vi "Sensor Loop.vi"() -> ()   [LabVIEW 2014, in "Elevator System.lvlib"]
uses:
  Elevator System.lvlib
  Typedef/FGVAction.ctl
  SimulatorVIs/Simulation Input Global.vi
  <vilib>/ptbypt/NI_PtbyPt.lvlib
panel:
  in  "elevators parameters":T1={"static gain"=10.0, "lag (s)"=0.05, "deadtime (s)"=0.01, "load"=0.0, "deadband"=0.0, "sensor noise"=0.0, "initial PV"=6.0, "plant noise"=0.0} {"plant noise" format="%.2f"; "initial PV" format="%.2f"; "sensor noise" format="%.2f"; "lag (s)" format="%.2f"; "deadtime (s)" format="%.2f"; "deadband" format="%.1f"; "load" format="%.2f"; "static gain" format="%.2f"}
  in  "gripper parameters":T1={"static gain"=2.5, "lag (s)"=2.5, "deadtime (s)"=0.01, "load"=40.0, "deadband"=0.0, "sensor noise"=0.0, "initial PV"=0.0, "plant noise"=0.0} {"plant noise" format="%.2f"; "initial PV" format="%.2f"; "sensor noise" format="%.2f"; "lag (s)" format="%.2f"; "deadtime (s)" format="%.2f"; "deadband" format="%.1f"; "load" format="%.2f"; "static gain" format="%.2f"}
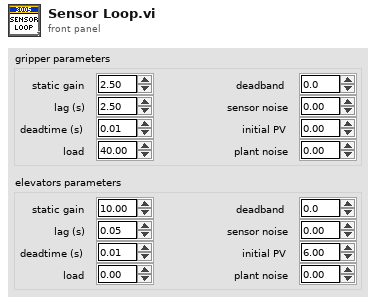
[diagram p1: front panel]
types:
  T1 = cluster{"static gain":dbl, "lag (s)":dbl, "deadtime (s)":dbl, "load":dbl, "deadband":dbl, "sensor noise":dbl, "initial PV":dbl, "plant noise":dbl}
  T2 = typedef "Elevator System.lvlib/FGVAction.ctl" = enum16{"get", "set"}
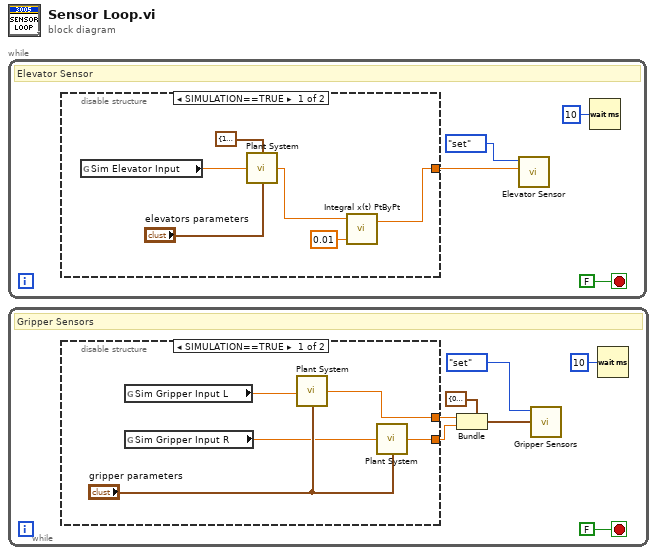
[diagram p0: block diagram]
diagram:
  n1 = while {
    stop <- FALSE stop-if-true
    # "Elevator Sensor"
    n2 = disable-structure shown="SIMULATION==TRUE" {
      disable-tunnel: [w6 _] -> w1
      frame condition #0 (active) {
        n3 = global read "Simulation Input Global.vi" "Sim Elevator Input"() -> (w9:dbl)
        n4 = call "Plant System.vi"("output saturation range"=cluster{"output high":dbl, "output low":dbl} {"output high"=100.0, "output low"=-100.0}, "Plant Input"=w9, "process parameters"="elevators parameters") -> ("Plant Output"=w7:dbl)  [unwired: 12 in]
        n5 = call <vilib>:"Integral x(t) PtByPt.vi"("dt"=0.01, "x"=w7) -> ("integral x(t)"=w6:dbl)  [unwired: 2 in, 1 out]
      }
      frame condition #1 {
      }
    }
    n6 = call "Elevator Sensor.vi"("Value"=w1, "Action"=FGVAction."set") -> ()  [unwired: 8 in, 2 out]
    n7 = Wait (ms)(milliseconds to wait=u32 10) -> ()  [unwired: 1 out]
  }
  n8 = while {
    stop <- FALSE stop-if-true
    # "Gripper Sensors"
    n9 = disable-structure shown="SIMULATION==TRUE" {
      disable-tunnel: [w19 _] -> w14
      disable-tunnel: [w18 _] -> w13
      frame condition #0 (active) {
        n10 = global read "Simulation Input Global.vi" "Sim Gripper Input L"() -> (w21:dbl)
        n11 = global read "Simulation Input Global.vi" "Sim Gripper Input R"() -> (w20:dbl)
        n12 = call "Plant System.vi"("Plant Input"=w21, "process parameters"="gripper parameters") -> ("Plant Output"=w19:dbl)  [unwired: 13 in]
        n13 = call "Plant System.vi"("Plant Input"=w20, "process parameters"="gripper parameters") -> ("Plant Output"=w18:dbl)  [unwired: 13 in]
      }
      frame condition #1 {
      }
    }
    n14 = Bundle(cluster=cluster{"Left":dbl, "Right":dbl} {"Left"=0.0, "Right"=0.0} ("Gripper Values"), "Left"=w14, "Right"=w13) -> (w11:cluster{"Left":dbl, "Right":dbl})
    n15 = call "Gripper Sensors.vi"("Input"=w11, "Action"=FGVAction."set") -> ()  [unwired: 8 in, 2 out]
    n16 = Wait (ms)(milliseconds to wait=u32 10) -> ()  [unwired: 1 out]
  }
